vi "Get Image Of VIs.vi"(4 "# of Columns":i32, 6 "# of Rows":i32, 8 "error in (no error)":errorcluster, 9 "Cell Bounds":T3, 11 "All VI Data":T1[](array[typedef])) -> (0 "error out":errorcluster, 3 "2D Picture":picture)   [LabVIEW 2011]
doc: "This VI will startup a clone for each element in <B>All VI Data</B>. This clone will display an image of the VI and the name of the VI.\n\nDeveloped by Brian Hoover brian@brian-hoover.com"
uses:
  <vilib>/Utility/miscctls.llb/LVBoundsTypeDef.ctl
  VI Data Type.ctl
  <vilib>/picture/picture.llb/imagedata.ctl
  <vilib>/Utility/miscctls.llb/LVRectTypeDef.ctl
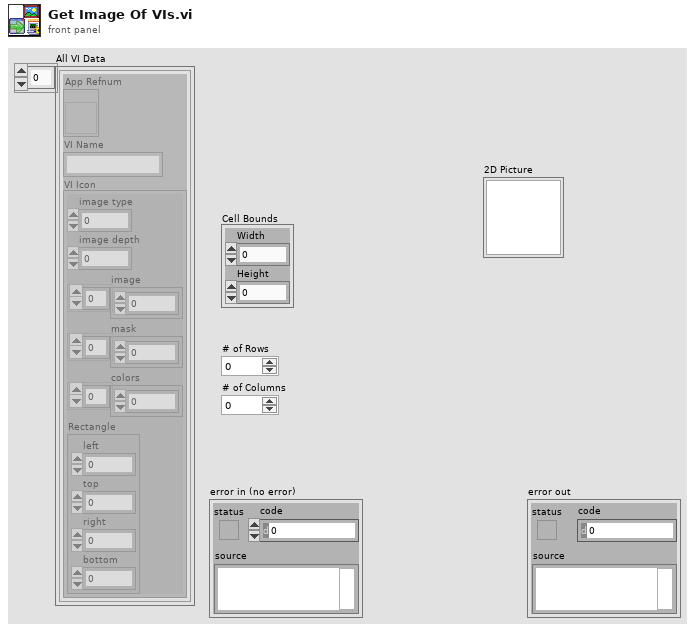
[diagram p1: front panel]
types:
  T1 = typedef "VI Data Type.ctl" = cluster{"App Refnum":refnum<vi>, "VI Name":string, "VI Icon":T2}
  T2 = typedef "imagedata.ctl" = cluster{"image type":i32, "image depth":i32, "image":u8[], "mask":u8[], "colors":u32[], "Rectangle":cluster{"left":i16, "top":i16, "right":i16, "bottom":i16}}
  T3 = typedef "LVBoundsTypeDef.ctl" = cluster{"Width":u32, "Height":u32}
  T4 = typedef "LVRectTypeDef.ctl" = cluster{"Left":i16, "Top":i16, "Right":i16, "Bottom":i16}
  T5 = cluster{"left":i16, "top":i16, "right":i16, "bottom":i16}
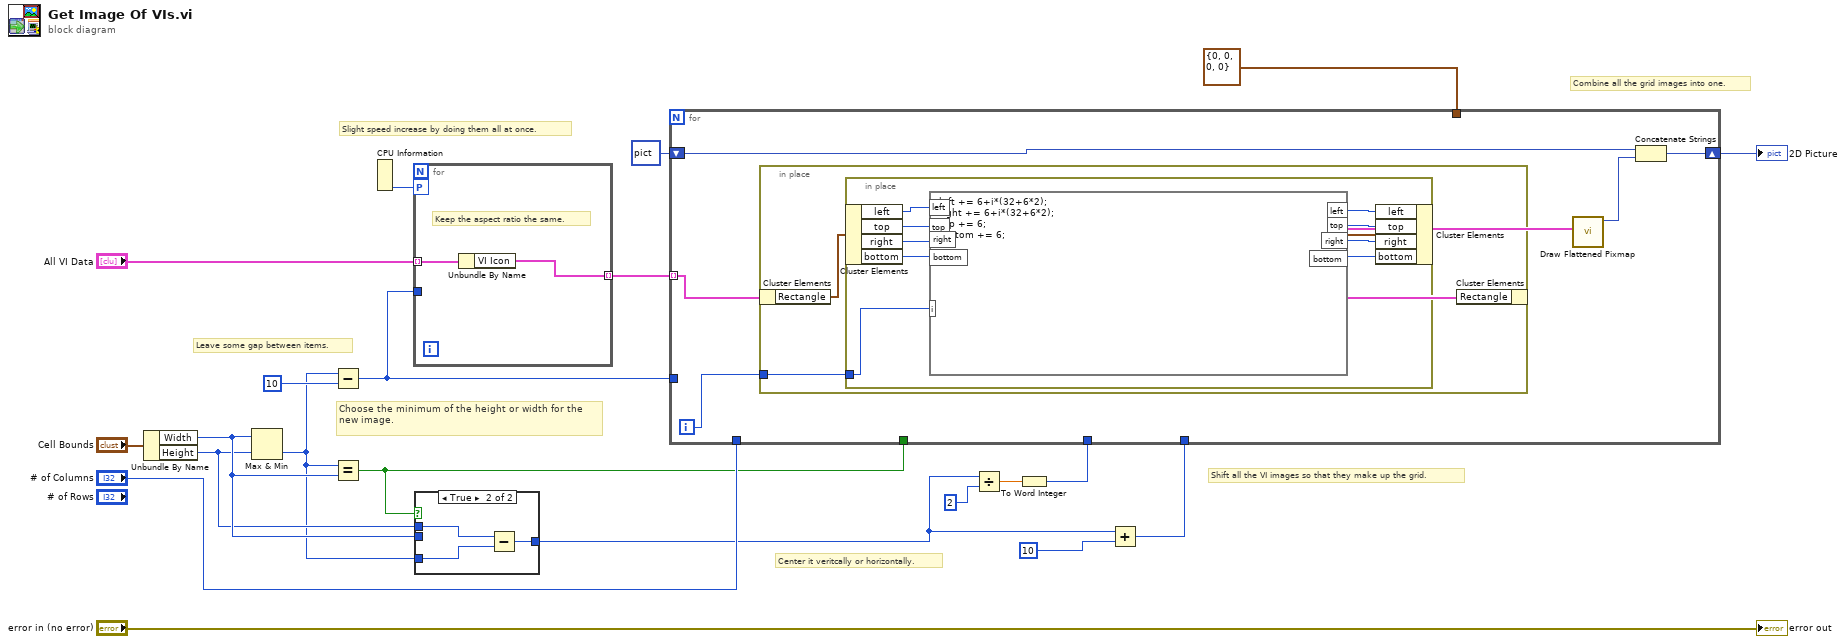
[diagram p0: block diagram]
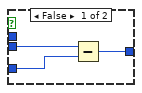
[diagram p2: hidden frame]
diagram:
  # "Center it veritcally or horizontally."
  # "Leave some gap between items."
  # "Choose the minimum of the height or width for the new image."
  # "Combine all the grid images into one."
  # "Shift all the VI images so that they make up the grid."
  # "Slight speed increase by doing them all at once."
  n1 = Unbundle By Name("Cell Bounds") -> ("Width"=w20:u32, "Height"=w19:u32)
  n2 = Max & Min(x=w20, y=w19) -> (min(x,y)=w10:u32)  [unwired: 1 out]
  n3 = Subtract(x=w10, y=10) -> (x-y=w12:u32)
  n4 = Equal?(x=w10, y=w20) -> (x = y?=w9:bool)
  n5 = CPU Information() -> (7:w1:i32)  [unwired: 3 out]
  n6 = for {
    tunnel: "All VI Data" -> [w23] mode=indexing
    tunnel: w12 -> [_]
    tunnel: [w22] -> w14 mode=indexing
    workers-P: w1 -> [_]
    # "Keep the aspect ratio the same."
    n7 = Unbundle By Name(w23) -> ("VI Icon"=w22:T2)
  }
  n8 = case shown="True" w9 {
    tunnel: w10 -> [w24 w29]
    tunnel: w19 -> [_ w28]
    tunnel: w20 -> [w25 _]
    tunnel: [w26 w27] -> w8
    frame False {
      n9 = Subtract(x=w25, y=w24) -> (x-y=w26:u32)
    }
    frame True {
      n10 = Subtract(x=w28, y=w29) -> (x-y=w27:u32)
    }
  }
  n11 = Divide(x=w8, y=u32 2) -> (x/y=w6:dbl)
  n12 = To Word Integer(number=w6) -> (16bit integer=w5:i16)
  n13 = Add(x=w8, y=u32 10 ("x")) -> (x+y=w4:u32)
  n14 = for {
    tunnel: w14 -> [w32] mode=indexing
    tunnel: w12 -> [_]
    tunnel: T4 {"Left"=0, "Top"=0, "Right"=0, "Bottom"=0} ("Front Panel Window:Window Bounds") -> [_]
    tunnel: "# of Columns" -> [_]
    tunnel: w9 -> [_]
    tunnel: w4 -> [_]
    tunnel: w5 -> [_]
    shift-right: [w34] -> w16
    shift-left: picture data[5B] -> [w33]
    i -> [w31]
    n15 = in-place {
      in-place-border: w31 -> [w37]
      n16 = in-place-cluster #1(w32) -> ("Rectangle"=w38:T5)
      n17 = in-place {
        in-place-border: w37 -> [w39]
        n18 = in-place-cluster #2(w38) -> ("left"=w47:i16, "top"=w46:i16, "right"=w45:i16, "bottom"=w44:i16)
        n19 = formula code="left += 6+i*(32+6*2);\nright += 6+i*(32+6*2);\ntop += 6;\nbottom += 6;"("left"=w47, "top"=w46, "right"=w45, "bottom"=w44, "i"=w39) -> ("left"=w43:i16, "top"=w42:i16, "right"=w41:i16, "bottom"=w40:i16)
        n20 = in-place-cluster #2("left"=w43, "top"=w42, "right"=w41, "bottom"=w40) -> (w36:T5)
      }
      n21 = in-place-cluster #1("Rectangle"=w36) -> (w30:T2)
    }
    n22 = call <vilib>:"Draw Flattened Pixmap.vi"("image data"=w30) -> ("new picture"=w35:picture)  [unwired: 8 in]
    n23 = Concatenate Strings(w33, w35) -> (w34:picture)
  }
  "2D Picture" <- w16
  "error out" <- "error in (no error)"
